vi "Vin_Vout_2C.vi"(4 "Fondo Scala AI1 (33)":dbl(ring)=10.0 items=["10"=10.0, "5"=5.0, "0.5"=0.5, "0.05"=0.05], 5 "Fondo Scala AI0 (68)":dbl(ring)=10.0 items=["10"=10.0, "5"=5.0, "0.5"=0.5, "0.05"=0.05], 6 "V in volt":dbl format="%0.2f", 7 "Canale uscita":tag="Dev1/ao0") -> (0 "sd 1":dbl format="%.5f", 1 "V1 medio":dbl format="%.5f", 2 "sd 0":dbl format="%.5f", 3 "V0 medio":dbl format="%.5f")   [LabVIEW 2014]
uses:
  <vilib>/DAQmx/write.llb/DAQmx Write (Analog DBL 1Chan 1Samp).vi
  <vilib>/DAQmx/read.llb/DAQmx Read (Analog 2D DBL NChan NSamp).vi
  <vilib>/DAQmx/create/channels.llb/DAQmx Create Channel (AO-Voltage-Basic).vi
  <vilib>/DAQmx/configure/timing.llb/DAQmx Timing (Sample Clock).vi
  <vilib>/DAQmx/miscellaneous.llb/DAQmx Fill In Error Info.vi
  <vilib>/DAQmx/create/channels.llb/DAQmx Create Channel (AI-Voltage-Basic).vi
  <vilib>/Analysis/NI_AALBase.lvlib
panel:
  # "RSE: 68 \nRSE: 33"
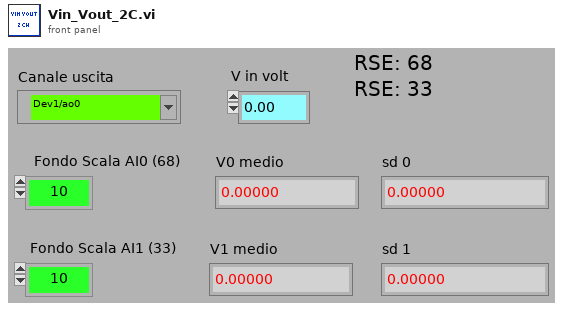
[diagram p1: front panel]
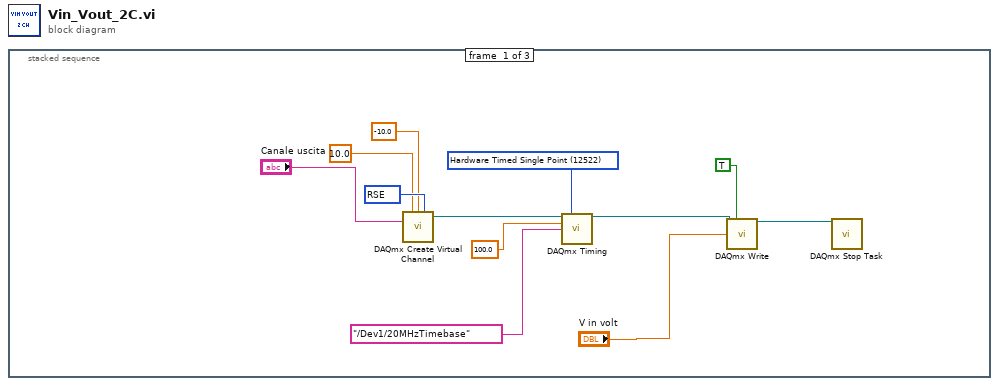
[diagram p0: block diagram]
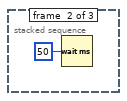
[diagram p2: hidden frame]
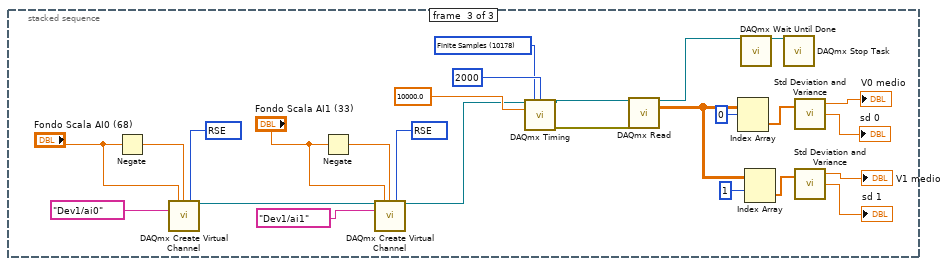
[diagram p3: hidden frame]
diagram:
  n1 = stacked-sequence {
    frame #0 {
      w8 = 12522 items=["Finite Samples"=10178, "Continuous Samples"=10123, "Hardware Timed Single Point"=12522] ("sample mode")
      w12 = 10083 items=["Default"=-1, "RSE"=10083, "Differential"=10106, "Pseudodifferential"=12529] ("output terminal configuration")
      n2 = call-poly <vilib>:"DAQmx Create Virtual Channel.vi"("maximum value"=10.0, "minimum value"=-10.0, "output terminal configuration"=w12, "physical channels"="Canale uscita") -> ("task out"=w4:refnum<k21>)  [unwired: 5 in, 6 out]
      n3 = call-poly <vilib>:"DAQmx Timing.vi"("task/channels in"=w4, "sample mode"=w8, "rate"=100.0, "source"=tag "/Dev1/20MHzTimebase") -> ("task out"=w6:refnum<k21>)  [unwired: 3 in, 8 out]
      n4 = call-poly <vilib>:"DAQmx Write.vi"("task/channels in"=w6, "auto start"=TRUE, "data"="V in volt") -> ("task out"=w5:refnum<k21>)  [unwired: 1 in, 11 out]
      n5 = call <vilib>:"DAQmx Stop Task.vi"("task/channels in"=w5) -> ()  [unwired: 1 in, 14 out]
    }
    frame #1 {
      n6 = Wait (ms)(milliseconds to wait=u32 50) -> ()  [unwired: 1 out]
    }
    frame #2 {
      w25 = 10083 items=["default"=-1, "RSE"=10083, "NRSE"=10078, "Differential"=10106, "Pseudodifferential"=12529] ("input terminal configuration")
      w31 = 10178 items=["Finite Samples"=10178, "Continuous Samples"=10123, "Hardware Timed Single Point"=12522] ("sample mode")
      w38 = 10083 items=["default"=-1, "RSE"=10083, "NRSE"=10078, "Differential"=10106, "Pseudodifferential"=12529] ("input terminal configuration")
      n7 = Negate(x="Fondo Scala AI0 (68)") -> (-x=w39:dbl)
      n8 = call-poly <vilib>:"DAQmx Create Virtual Channel.vi"("maximum value"="Fondo Scala AI0 (68)", "minimum value"=w39, "input terminal configuration"=w38, "physical channels"=tag "Dev1/ai0") -> ("task out"=w22:refnum<k21>)  [unwired: 5 in, 6 out]
      n9 = Negate(x="Fondo Scala AI1 (33)") -> (-x=w26:dbl)
      n10 = call-poly <vilib>:"DAQmx Create Virtual Channel.vi"("task in"=w22, "maximum value"="Fondo Scala AI1 (33)", "minimum value"=w26, "input terminal configuration"=w25, "physical channels"=tag "Dev1/ai1") -> ("task out"=w21:refnum<k21>)  [unwired: 4 in, 6 out]
      n11 = call-poly <vilib>:"DAQmx Timing.vi"("task/channels in"=w21, "sample mode"=w31, "samples per channel"=u32 2000, "rate"=10000.0) -> ("task out"=w36:refnum<k21>, "error out"=w35:errorcluster)  [unwired: 3 in, 7 out]
      n12 = call-poly <vilib>:"DAQmx Read.vi"("task/channels in"=w36, "error in"=w35) -> ("task out"=w32:refnum<k21>, "data"=w16:dbl[][])  [unwired: 1 in, 11 out]
      n13 = Index Array(array=w16, index (row)=0 ("index")) -> (element=w15:dbl[])  [unwired: 1 in]
      n14 = call <vilib>:"DAQmx Wait Until Done.vi"("task/channels in"=w32) -> ("task out"=w30:refnum<k21>)  [unwired: 2 in, 12 out]
      n15 = Index Array(array=w16, index (row)=1 ("index")) -> (element=w14:dbl[])  [unwired: 1 in]
      n16 = call <vilib>:"DAQmx Stop Task.vi"("task/channels in"=w30) -> ()  [unwired: 1 in, 14 out]
      n17 = call <vilib>:"Std Deviation and Variance.vi"("X"=w15) -> ("mean"=→"V0 medio":dbl, "standard deviation"=→"sd 0":dbl)  [unwired: 1 in, 1 out]
      n18 = call <vilib>:"Std Deviation and Variance.vi"("X"=w14) -> ("mean"=→"V1 medio":dbl, "standard deviation"=→"sd 1":dbl)  [unwired: 1 in, 1 out]
    }
  }
